vi "p6vision estereo.vi"() -> ()   [LabVIEW 2017]
panel:
  out "Z":dbl
  out "F":dbl
  in  "Z":dbl
  in  "F":dbl
  in  "O":dbl
  in  "Enum 2":enum16{"calibrar", "medir distancia"}(ring)
  in  "Enum":enum16{"no guardar", "izquierda", "derecha"}(ring)
  out "new picture 2":picture
  in  "Slide 2":dbl(slide) scale=0.0..255.0
  out "Array":dbl[](array[numeric])
  out "Image Out":T1(plugin-control)
  out "x":dbl
  out "y":dbl
  in  "Stop (F)":bool
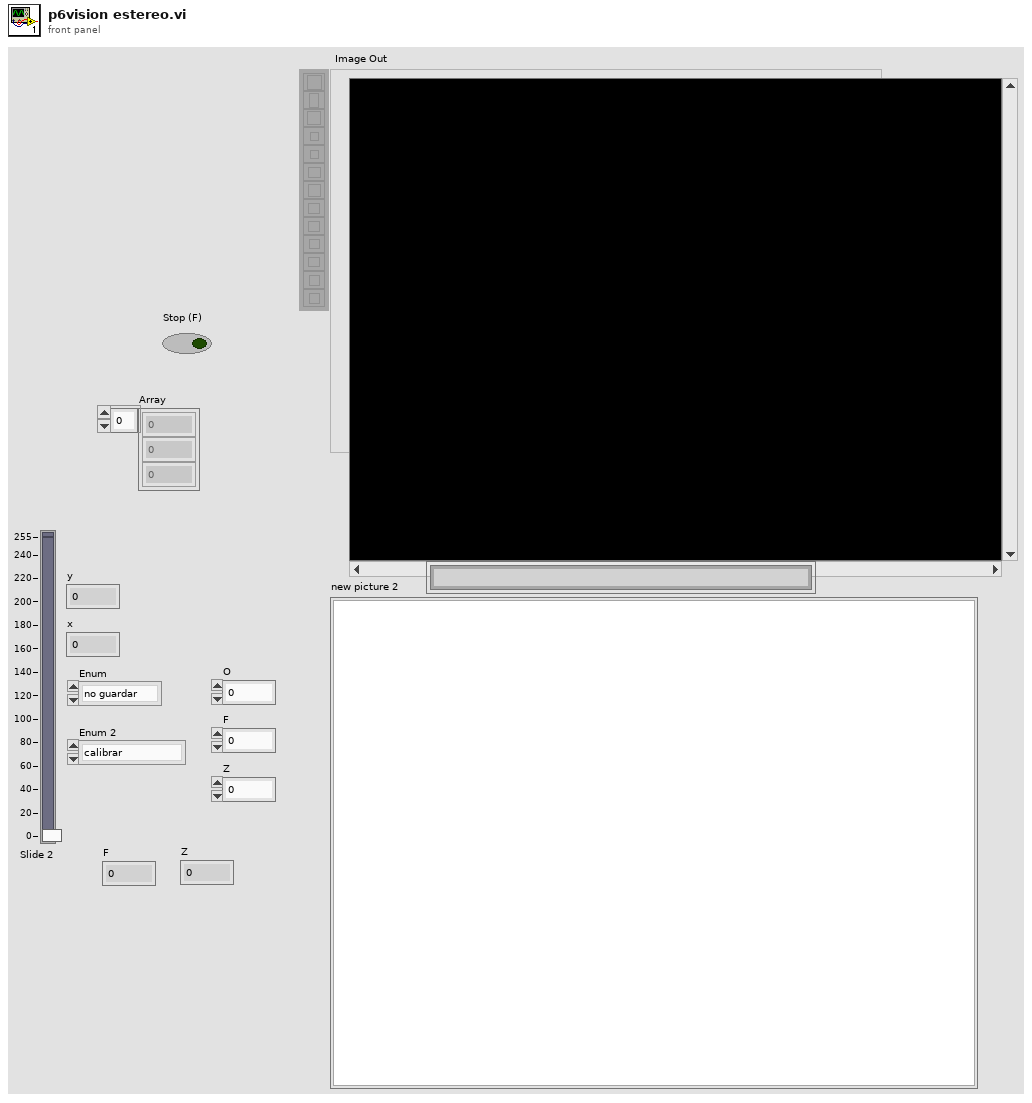
[diagram p1: front panel]
types:
  T1 = typedef "IMAQ Image.ctl" = refnum<image>
  T2 = typedef "imagedata.ctl" = cluster{"image type":i32, "image depth":i32, "image":u8[], "mask":u8[], "colors":u32[], "Rectangle":cluster{"left":i16, "top":i16, "right":i16, "bottom":i16}}
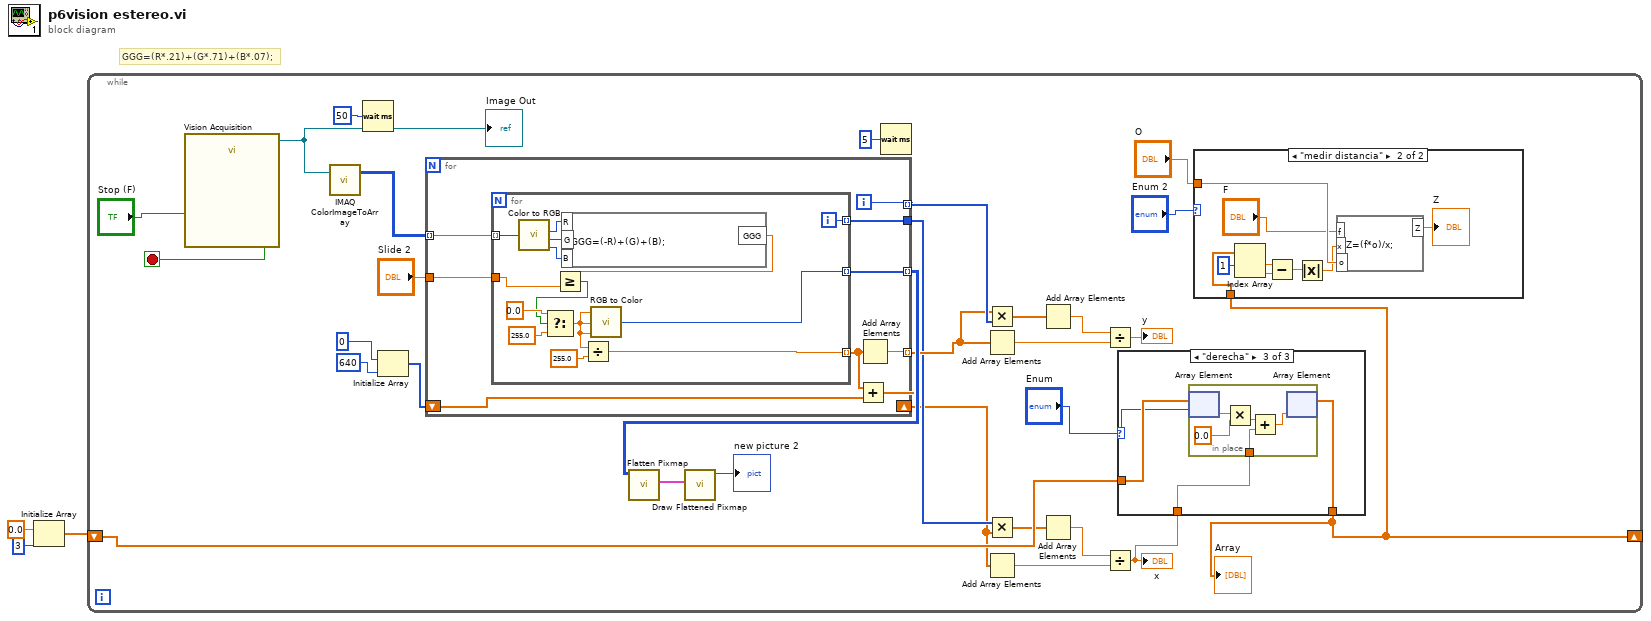
[diagram p0: block diagram]
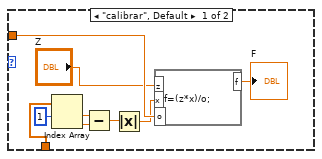
[diagram p2: hidden frame]
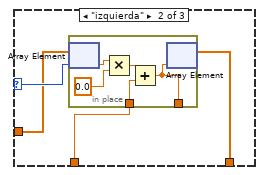
[diagram p4: hidden frame]
diagram:
  # "GGG=(R*.21)+(G*.71)+(B*.07);"
  n1 = Initialize Array(0.0 ("element"), 3 ("dimension size")) -> (w3:dbl[])
  n2 = while {
    shift-right: [w5] -> _
    shift-left: w3 -> [w24]
    stop <- w33 stop-if-true
    n3 = call "Vision Acquisition"("Stop (F)"="Stop (F)") -> ("Image Out"=w32:T1, "Stopped"=w33:bool)  [unwired: 24 in, 1 out]
    "Image Out" <- w32
    n4 = call "IMAQ ColorImageToArray"("Image"=w32) -> ("Image Pixels (U32)"=w16:u32[][])  [unwired: 3 in, 2 out]
    n5 = Wait (ms)(milliseconds to wait=u32 50) -> ()  [unwired: 1 out]
    n6 = Initialize Array(0 ("element"), 640 ("dimension size")) -> (w21:i32[])
    n7 = for {
      tunnel: w16 -> [w60] mode=indexing
      tunnel: "Slide 2" -> [w59]
      tunnel: [w58] -> w12 mode=indexing
      tunnel: [w57] -> w13 mode=indexing
      shift-right: [w54] -> w10
      shift-left: w21 -> [w55]
      tunnel: [w53] -> w11
      tunnel: [w52] -> w19 mode=indexing
      i -> [w57]
      n8 = for {
        tunnel: w60 -> [w66] mode=indexing
        tunnel: w59 -> [w72]
        tunnel: [w70] -> w56 mode=indexing
        tunnel: [w69] -> w53 mode=indexing
        tunnel: [w63] -> w52 mode=indexing
        i -> [w69]
        n9 = call <vilib>:"Color to RGB.vi"("Color"=w66) -> ("R"=w62:u8, "G"=w68:u8, "B"=w67:u8)  [unwired: 1 out]
        n10 = formula code="GGG=(-R)+(G)+(B);"("R"=w62, "G"=w68, "B"=w67) -> ("GGG"=w61:dbl)
        n11 = Greater Or Equal?(x=w61, y=w72) -> (x >= y?=w65:bool)
        n12 = Select(t=0.0, s=w65, f=255.0) -> (s? t:f=w64:dbl)
        n13 = Divide(x=w64, y=255.0) -> (x/y=w70:dbl)
        n14 = call <vilib>:"RGB to Color.vi"("B"=w64, "G"=w64, "R"=w64) -> ("Color"=w63:u32)
      }
      n15 = Add(x=w56, y=w55) -> (x+y=w54:dbl[])
      n16 = Add Array Elements(numeric array=w56) -> (sum=w58:dbl)
    }
    n17 = call <vilib>:"Flatten Pixmap.vi"("24-bit pixmap"=w19) -> ("image data"=w18:T2)  [unwired: 10 in]
    n18 = call <vilib>:"Draw Flattened Pixmap.vi"("image data"=w18) -> ("new picture"=→"new picture 2":picture)  [unwired: 8 in]
    n19 = Wait (ms)(milliseconds to wait=u32 5) -> ()  [unwired: 1 out]
    n20 = Multiply(x=w12, y=w13) -> (x*y=w8:dbl[])
    n21 = Add Array Elements(numeric array=w12) -> (sum=w30:dbl)
    n22 = Multiply(x=w11, y=w10) -> (x*y=w9:dbl[])
    n23 = Add Array Elements(numeric array=w10) -> (sum=w29:dbl)
    n24 = Add Array Elements(numeric array=w8) -> (sum=w31:dbl)
    n25 = Add Array Elements(numeric array=w9) -> (sum=w28:dbl)
    n26 = Divide(x=w31, y=w30) -> (x/y=→"y":dbl)
    n27 = Divide(x=w28, y=w29) -> (x/y=w23:dbl)
    "x" <- w23
    n28 = case shown="\"derecha\"" "Enum" {
      selector: "Enum" -> [_ w79 w87]
      tunnel: w24 -> [w75 w78 w88]
      tunnel: [w75 w76 w85] -> w5
      tunnel: w23 -> [_ w77 w86]
      frame "no guardar", Default {
      }
      frame "izquierda" {
        n29 = in-place {
          in-place-border: w77 -> [w84]
          in-place-border: [w80] -> _
          n30 = in-place-array #1(w78, w79) -> (w83:dbl)
          n31 = Multiply(x=w83, y=0.0) -> (x*y=w81:dbl)
          n32 = Add(x=w81, y=w84) -> (x+y=w80:dbl)
          n33 = in-place-array #1(w80) -> (w76:dbl[])  [unwired: 1 out]
        }
      }
      frame "derecha" {
        n34 = in-place {
          in-place-border: w86 -> [w90]
          n35 = in-place-array #2(w88, w87) -> (w93:dbl)
          n36 = Multiply(x=w93, y=0.0) -> (x*y=w91:dbl)
          n37 = Add(x=w91, y=w90) -> (x+y=w89:dbl)
          n38 = in-place-array #2(w89) -> (w85:dbl[])  [unwired: 1 out]
        }
      }
    }
    "Array" <- w5
    n39 = case shown="\"medir distancia\"" "Enum 2" {
      tunnel: w5 -> [w41 w47]
      tunnel: "O" -> [w37 w46]
      frame "calibrar", Default {
        n40 = Index Array(array=w41, index #1=1 ("index")) -> (element #1=w39:dbl, element #2=w40:dbl)  [unwired: 1 in]
        n41 = Subtract(x=w39, y=w40) -> (x-y=w38:dbl)
        n42 = Absolute Value(x=w38) -> (abs(x)=w35:dbl)
        n43 = formula code="f=(z*x)/o;"("z"="Z", "x"=w35, "o"=w37) -> ("f"=→"F":dbl)
      }
      frame "medir distancia" {
        n44 = Index Array(array=w47, index #1=1 ("index")) -> (element #1=w49:dbl, element #2=w50:dbl)  [unwired: 1 in]
        n45 = Subtract(x=w49, y=w50) -> (x-y=w48:dbl)
        n46 = Absolute Value(x=w48) -> (abs(x)=w45:dbl)
        n47 = formula code="Z=(f*o)/x;"("f"="F", "x"=w45, "o"=w46) -> ("Z"=→"Z":dbl)
      }
    }
  }
